vi "EMBALLAGE_BDD_rechercheImprimantes.vi"() -> ()   [LabVIEW 2019]
panel:
  out "Tableau":string[](array[string])
  out "nom":string[](array[string])
  out "tableau":string[][](array[string])
  out "error out":errorcluster caption="sortie d'erreur"
  out "standard error":string caption="erreur standard"
  out "standard output":string caption="sortie standard"
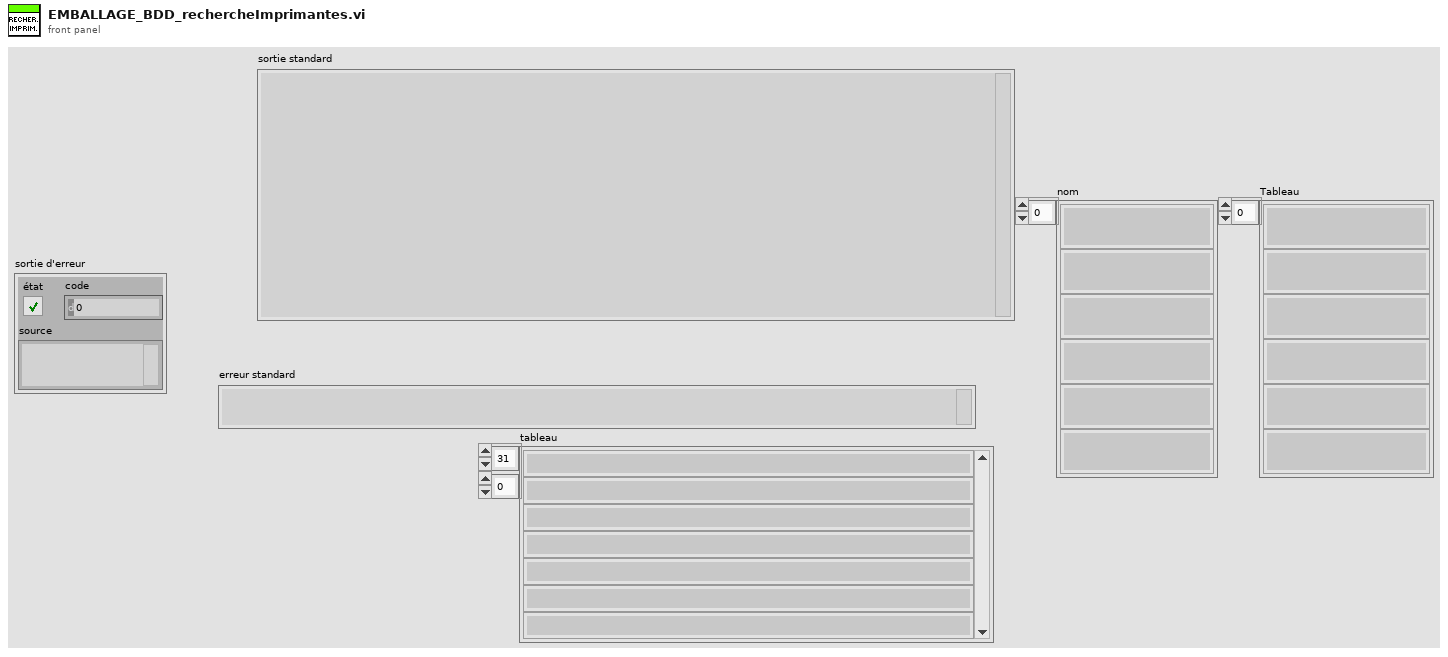
[diagram p1: front panel]
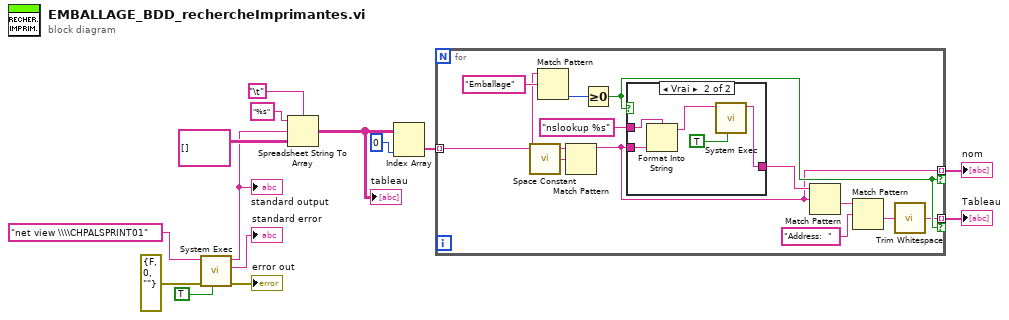
[diagram p0: block diagram]
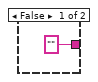
[diagram p2: hidden frame]
diagram:
  n1 = call <vilib>:"System Exec.vi"("run minimized? (F)"=TRUE, "error in (no error)"=errorcluster {"status"=FALSE, "code"=0, "source"=""}, "command line"="net view \\\\CHPALSPRINT01") -> ("error out"=→"error out":errorcluster, "standard error"=→"standard error":string, "standard output"=w6:string)  [unwired: 5 in, 1 out]
  "standard output" <- w6
  n2 = Spreadsheet String To Array(delimiter (Tab)="\t", format string="%s" ("chaîne de format"), spreadsheet string=w6, array type (2D Dbl)=string[][] []) -> (array=w1:string[][])
  "tableau" <- w1
  n3 = Index Array(array=w1, index (col)=0 ("indice désactivé (col)")) -> (element=w4:string[])  [unwired: 1 in]
  n4 = for {
    tunnel: w4 -> [w24] mode=indexing
    tunnel: [w19] -> w5 mode=indexing if=w21
    tunnel: [w15] -> w2 mode=indexing if=w21
    n5 = call <vilib>:"Space Constant.vi"() -> ("String"=w23:string)
    n6 = Match Pattern(string=w24, regular expression="Emballage" ("expression régulière")) -> (offset past match=w25:i32)  [unwired: 1 in, 3 out]
    n7 = Match Pattern(string=w24, regular expression=w23) -> (before substring=w19:string)  [unwired: 1 in, 3 out]
    n8 = Greater Or Equal To 0?(x=w25) -> (x >= 0?=w21:bool)
    n9 = case shown="Vrai" w21 {
      tunnel: "nslookup %s" ("chaîne de format") -> [_ w32]
      tunnel: w19 -> [_ w31]
      tunnel: ["" ("standard output") w29] -> w20
      frame False {
      }
      frame True {
        n10 = Format Into String(format string=w32, w31) -> (resulting string=w30:string)  [unwired: 2 in, 1 out]
        n11 = call <vilib>:"System Exec.vi"("run minimized? (F)"=TRUE, "command line"=w30) -> ("standard output"=w29:string)  [unwired: 6 in, 3 out]
      }
    }
    n12 = Match Pattern(string=w20, regular expression=w19) -> (after substring=w18:string)  [unwired: 1 in, 3 out]
    n13 = Match Pattern(string=w18, regular expression="Address:  " ("expression régulière")) -> (after substring=w16:string)  [unwired: 1 in, 3 out]
    n14 = call <vilib>:"Trim Whitespace.vi"("string"=w16) -> ("trimmed string"=w15:string)  [unwired: 1 in]
  }
  "nom" <- w5
  "Tableau" <- w2
